vi "clientDetachBroadcast.vi"(8 "error in (no error)":errorcluster, 11 "SM1000-control in":T1) -> (0 "error out":errorcluster, 3 "SM1000-control out":T1)   [LabVIEW 2013, in "SLMControl.lvlib" / "SM1000.lvclass"]
doc: "Terminate the connection to the broadcast mechanism.\n\nThis method is used by a client application to terminate a connection to the broadcast mechanism of the EC1000."
uses:
  SM1000.lvclass
  Object-reference.ctl
  SM1000.lvclass/SM1000.ctl
  Custom-errors.ctl
  C:/Users/vangeste/Desktop/2015-06-02 - SLM - MAIF/HC-HardwareCharacterization/Sources/SM1000/LECBroadcast.dll
  HC-HardwareCharacterization/Sources/SM1000/LECBroadcast.dll
  DOTNET-error-int.vi
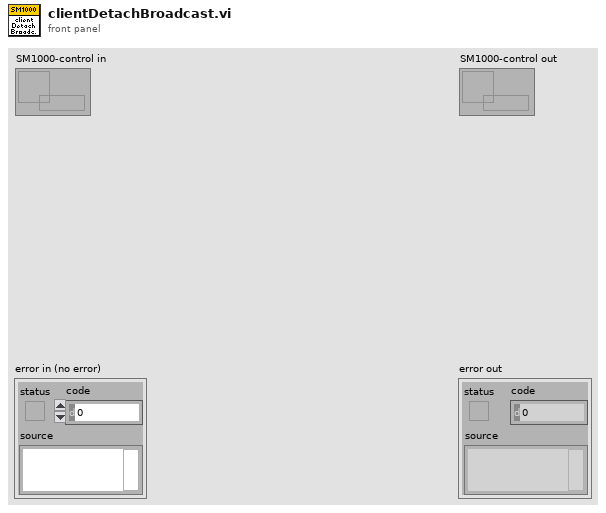
[diagram p1: front panel]
types:
  T1 = typedef "SLMControl.lvlib/SM1000.lvclass/Object-reference.ctl" = refnum<data-value>
  T2 = typedef "SLMControl.lvlib/SM1000.lvclass/Custom-errors.ctl" = enum16{"No error", "Not implemented", "Command not recognized", "Invalid input", "No connection", "Timeout", "Resource not loaded"}
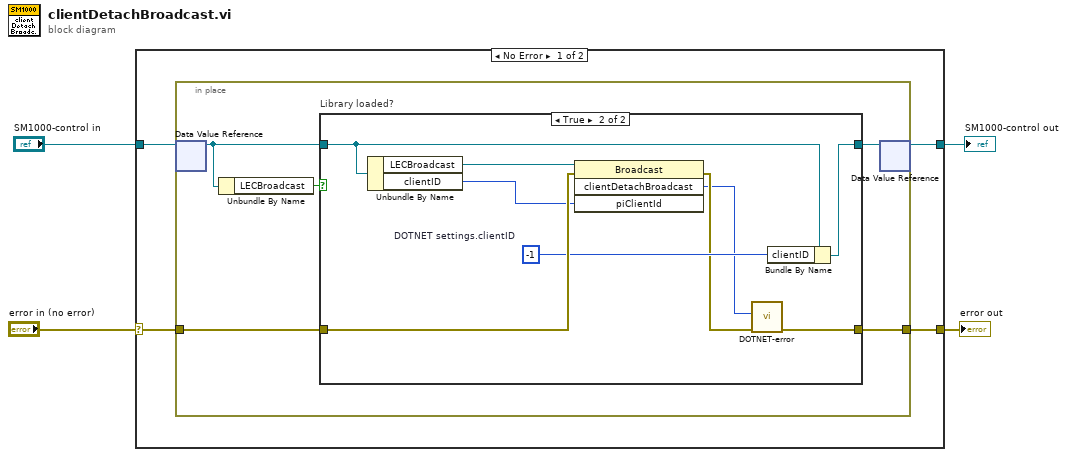
[diagram p0: block diagram]
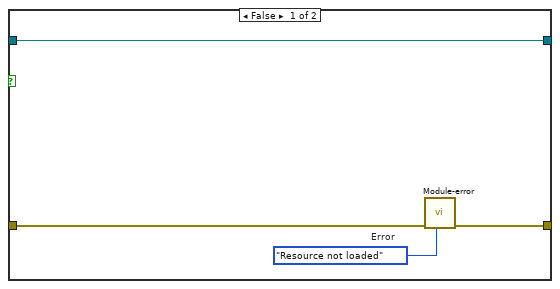
[diagram p2: hidden frame]
diagram:
  n1 = case shown="No Error" "error in (no error)" {
    selector: "error in (no error)" -> [w6 w28]
    tunnel: [w5 w28] -> w3
    tunnel: [w7 w27] -> w1
    tunnel: "SM1000-control in" -> [w8 w27]
    frame No Error {
      n2 = in-place {
        in-place-border: w6 -> [w13]
        in-place-border: [w10] -> w5
        n3 = in-place-dvr #1(w8) -> (w11:refnum<class "SM1000.lvclass">)  [unwired: 1 out]
        n4 = Unbundle By Name(w11) -> ("LECBroadcast"=w12:bool)
        n5 = case "Library loaded?" shown="True" w12 {
          tunnel: w13 -> [w17 w24]
          tunnel: w11 -> [w15 w26]
          tunnel: [w16 w20] -> w10
          tunnel: [w15 w23] -> w9
          frame False {
            w14 = Custom-errors."Resource not loaded"  # Error
            n6 = call "Module-error.vi"("Error"=w14, "error in (no error)"=w17) -> ("error out"=w16:errorcluster)  [unwired: 9 in]
          }
          frame True {
            w21 = -1  # DOTNET settings.clientID
            n7 = Unbundle By Name(w26) -> ("LECBroadcast"=w25:refnum<k24>, "clientID"=w22:i32)
            n8 = invoke class="Broadcast" method="clientDetachBroadcast"(reference=w25, error in=w24, "piClientId"=w22) -> (error out=w19:errorcluster, "clientDetachBroadcast"=w18:u32)  [unwired: 1 in, 2 out]
            n9 = call-poly "DOTNET-error.vi"("error in (no error)"=w19, "Retun code"=w18) -> ("error out"=w20:errorcluster)  [unwired: 9 in]
            n10 = Bundle By Name(cluster=w26, "clientID"=w21) -> (w23:refnum<class "SM1000.lvclass">)
          }
        }
        n11 = in-place-dvr #1(w9) -> (w7:T1)  [unwired: 1 out]
      }
    }
    frame Error {
    }
  }
  "error out" <- w3
  "SM1000-control out" <- w1
